vi "Programmatically Add Ring Items.vi"() -> ()   [LabVIEW 2023]
doc: "This example demonstrates the Menu Ring control, and how to programmatically add items to a ring."
panel:
  in  "Add New Ring Item":bool
  in  "New Ring Item Value":u32=1000000
  in  "New Ring Item Text":string="1 MHz"
  in  "Sample Rate":u32(ring)=10 items=["10 Hz"=10, "100 Hz"=100, "1 kHz"=1000]
  in  "Stop":bool
  # "Overview: Demonstrates the use of the Menu Ring control, and how to programmatically add items to the ring.\nInstructions:\n1. Run the VI.\n2. Change the value of the Sample Rate ring and notice its actual numeric value change in its digital display.\n3. Click the Add New Ring Item button to programmatically add a new item to the ring.\n4. Choose the <Other> option on the Ring to specify an undefined value via the digital display.\n5. Click Stop to stop the VI."
  # "New Ring Item"
  # "Right-click a ring and choose Visible Items > Digital Display to see the numeric value of the ring."
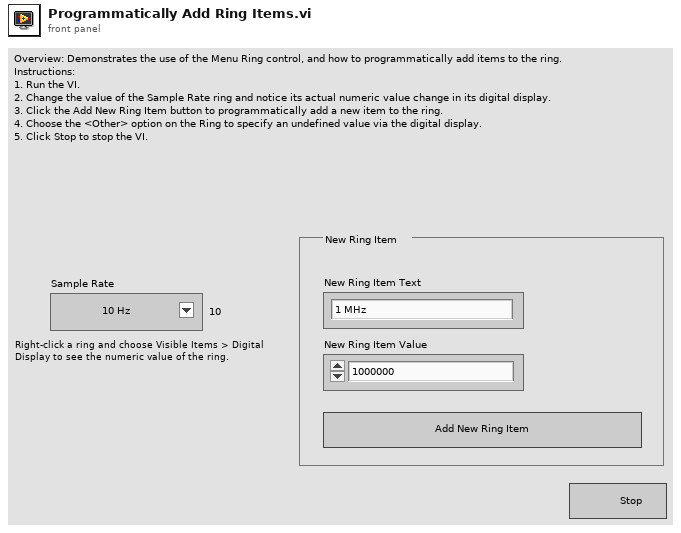
[diagram p1: front panel]
types:
  T1 = typedef "LVStringsAndValuesArrayTypeDef_U32.ctl" = cluster{"String":string, "Value":u32}[]
  T2 = cluster{"New Ring Item Text":string, "New Ring Item Value":u32}
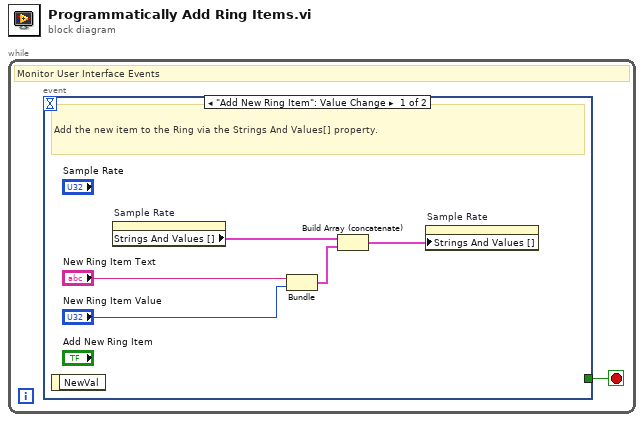
[diagram p0: block diagram]
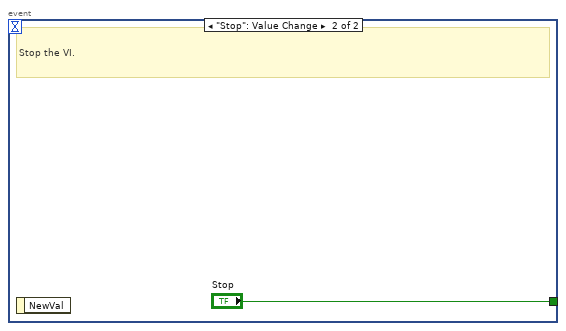
[diagram p2: hidden frame]
diagram:
  n1 = while {
    stop <- w1 stop-if-true
    # "Monitor User Interface Events"
    n2 = event shown="[0] \"Add New Ring Item\": Value Change" {
      selector: _ -> [_ _]
      dyn-events: _ -> [_ _]
      timeout: _ -> [_ _]
      tunnel: [_ "Stop"] -> w1
      event "Add New Ring Item": Value Change {
        # "Add the new item to the Ring via the Strings And Values[] property."
        n3 = event-data() -> ()  [unwired: 1 in, 1 out]
        n4 = property on="Sample Rate" class="Ring (strict)"() -> ("Strings And Values []"=w4:T1)  [unwired: 2 in, 2 out]
        n5 = Bundle("New Ring Item Text"="New Ring Item Text", "New Ring Item Value"="New Ring Item Value") -> (w6:T2)  [unwired: 1 in]
        n6 = Build Array (concatenate)(w4, w6) -> (w5:T1)
        n7 = property on="Sample Rate" class="Ring (strict)"("Strings And Values []"=w5) -> ()  [unwired: 2 in, 2 out]
      }
      event "Stop": Value Change {
        # "Stop the VI."
        n8 = event-data() -> ()  [unwired: 1 in, 1 out]
      }
    }
  }
